vi "LogToStringControl.vi"(4 "Reduce By (0.2)":dbl=0.2, 5 "Clear":bool, 6 "Reduce Every (100)":i32=100, 7 "Enable":bool=TRUE, 8 "Time Stamp (T/F or Format)":variant=variant(bool FALSE), 9 "Prefix (\"\")":string, 10 "Log Text (\"\")":string, 11 "String Ref":refnum<vi>) -> (3 "String Ref out":refnum<vi>)   [LabVIEW 2021]
uses:
  <vilib>/regexp/Match Regular Expression.xnode
  <vilib>/Utility/Data Type/NI_Data Type.lvlib
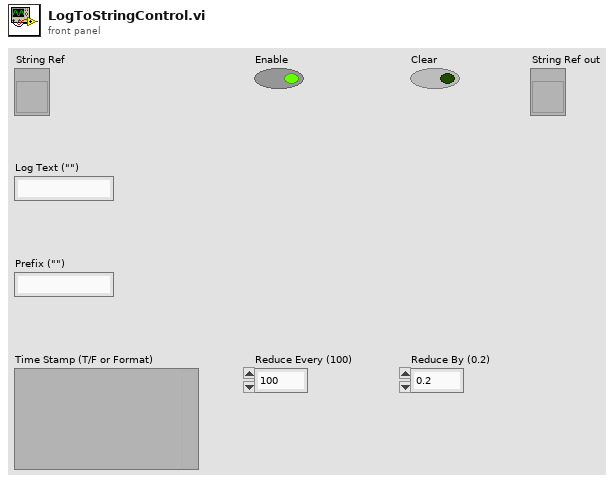
[diagram p1: front panel]
types:
  T1 = enum16{"Native", "Native Command Line", "UNIX", "Macintosh", "DOS"}
  T2 = typedef "NI_Data Type.lvlib/Data Type.ctl" = enum8{"Invalid Type", "Void", "I8", "I16", "I32", "I64", "U8", "U16", "U32", "U64", "Single Float", "Double Float", "Extended Float", "Single Complex", "Double Complex", "Extended Complex", "Enum U8", "Enum U16", "Enum U32", "Enum U64", "Single Float With Unit", "Double Float With Unit", "Extended Float With Unit", "Single Complex with Unit", "Double Complex with Unit", "Extended Complex with Unit", "Boolean", "String", "Path", "Picture", "Tag", "Array", "Cluster", "Variant", "LV Variant", "Waveform", "Timestamp", "Digital Waveform", "Digital Data", "ExpressData", "Refnum", "External Data", "VI", "Poly VI", "LabVIEW Class Instance", "Fixed Point", "Set Collection", "Map Collection"}
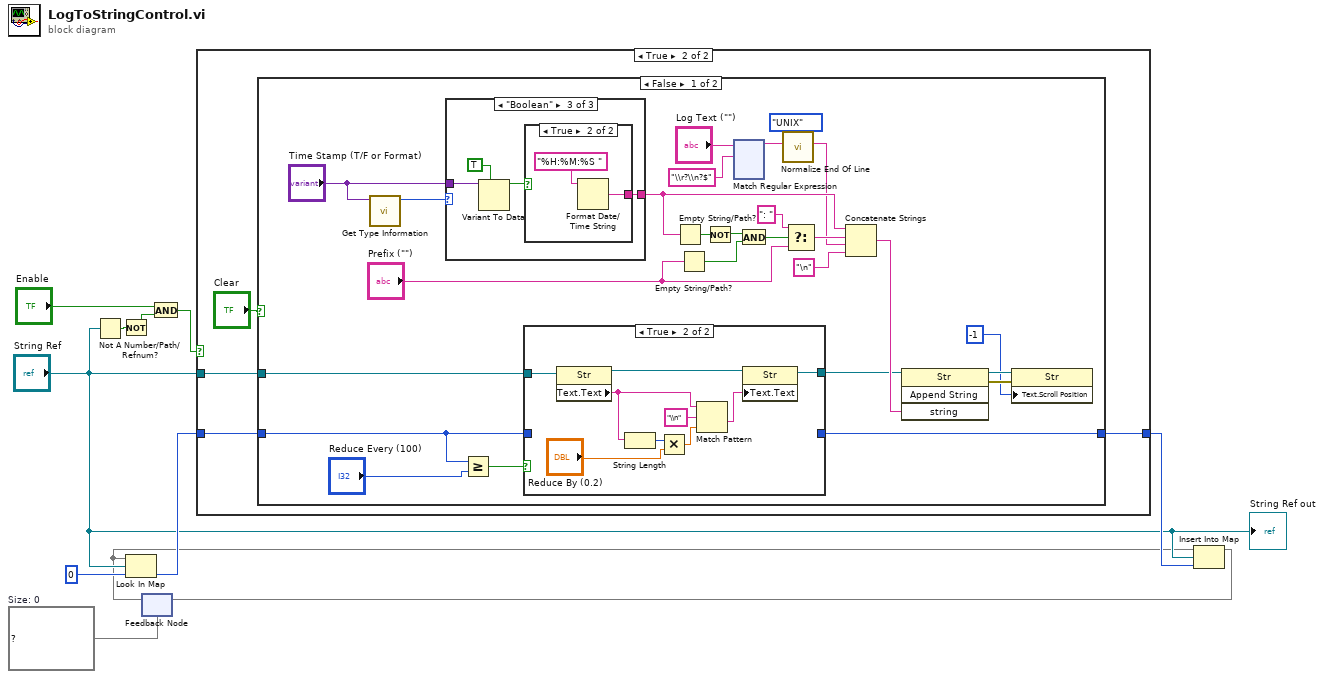
[diagram p0: block diagram]
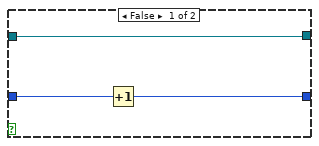
[diagram p3: hidden frame]
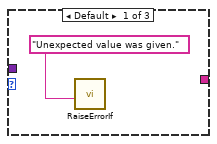
[diagram p4: hidden frame]
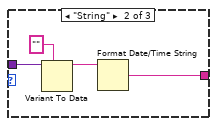
[diagram p5: hidden frame]
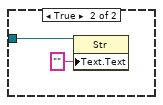
[diagram p7: hidden frame]
diagram:
  w7 = map{refnum<vi>, i32} {}  # Size: 0
  n1 = Not A Number/Path/Refnum?(number/path/refnum="String Ref") -> (NaN/Path/Refnum?=w10:bool)
  n2 = Not(x=w10) -> (.not. x?=w9:bool)
  n3 = feedback #1(w7) -> (w1:map{refnum<vi>, i32})
  n4 = Look In Map(map=w1, key="String Ref", default value=0) -> (value=w5:i32)  [unwired: 1 out]
  n5 = And(x="Enable", y=w9) -> (x .and. y?=w8:bool)
  n6 = case shown="True" w8 {
    tunnel: "String Ref" -> [_ w16]
    tunnel: w5 -> [w12 w15]
    tunnel: [w12 w14] -> w4
    frame False {
    }
    frame True {
      n7 = case shown="False" "Clear" {
        tunnel: w16 -> [w42 w184]
        tunnel: w15 -> [w26 _]
        tunnel: [w25 _] -> w14
        frame False {
          n8 = call <vilib>:"Get Type Information.vi"("variant"="Time Stamp (T/F or Format)") -> ("type"=w34:T2)  [unwired: 6 in, 4 out]
          n9 = case shown="\"Boolean\"" w34 {
            tunnel: "Time Stamp (T/F or Format)" -> [_ w175 w180]
            tunnel: [_ w173 w177] -> w40
            frame Default {
              n10 = call "RaiseErrorIf.vi"("error message"="Unexpected value was given.") -> ()  [unwired: 10 in, 1 out]
            }
            frame "String" {
              n11 = Variant To Data(type="" ("Log Text (\"\")"), Variant=w175) -> (data=w174:string)  [unwired: 1 in, 1 out]
              n12 = Format Date/Time String(time format string (%c)=w174) -> (date/time string=w173:string)  [unwired: 2 in]
            }
            frame "Boolean" {
              n13 = Variant To Data(type=TRUE, Variant=w180) -> (data=w178:bool)  [unwired: 1 in, 1 out]
              n14 = case shown="True" w178 {
                tunnel: [_ w181] -> w177
                frame False {
                }
                frame True {
                  n15 = Format Date/Time String(time format string (%c)="%H:%M:%S ") -> (date/time string=w181:string)  [unwired: 2 in]
                }
              }
            }
          }
          n16 = Greater Or Equal?(x=w26, y="Reduce Every (100)") -> (x >= y?=w32:bool)
          n17 = case shown="True" w32 {
            tunnel: w42 -> [w162 w171]
            tunnel: w26 -> [w161 _]
            tunnel: [w162 w163] -> w30
            tunnel: [w160 _] -> w25
            frame False {
              n18 = Increment(x=w161) -> (x+1=w160:i32)
            }
            frame True {
              n19 = property class="Str"(reference=w171) -> (reference out=w165:refnum<vi>, "Text.Text"=w166:string)  [unwired: 1 in, 1 out]
              n20 = String Length(string=w166) -> (length=w170:i32)
              n21 = Multiply(x=w170, y="Reduce By (0.2)") -> (x*y=w167:dbl)
              n22 = Match Pattern(string=w166, regular expression="\\n", offset (0)=w167) -> (after substring=w164:string)  [unwired: 3 out]
              n23 = property class="Str"(reference=w165, "Text.Text"=w164) -> (reference out=w163:refnum<vi>)  [unwired: 1 in, 1 out]
            }
          }
          n24 = Empty String/Path?(string/path=w40) -> (empty?=w35:bool)
          n25 = Empty String/Path?(string/path="Prefix (\"\")") -> (empty?=w39:bool)
          n26 = Not(x=w35) -> (.not. x?=w38:bool)
          n27 = xnode "Match Regular Expression"("input string"="Log Text (\"\")", "regular expression"="\\r?\\n?$") -> ("before match"=w18:string)  [unwired: 4 in, 4 out]
          n28 = And(x=w38, y=w39) -> (x .and. y?=w36:bool)
          n29 = call <vilib>:"Normalize End Of Line.vi"("end of line (Native)"=T1."UNIX", "string in"=w18) -> ("string out"=w22:string)  [unwired: 6 in]
          n30 = Select(t=": ", s=w36, f="Prefix (\"\")") -> (s? t:f=w41:string)
          n31 = Concatenate Strings(w40, w41, w22, "\n" ("string")) -> (w31:string)
          n32 = invoke class="Str" method="Append String"(reference=w30, "string"=w31) -> (reference out=w29:refnum<vi>, error out=w28:errorcluster)  [unwired: 2 in, 2 out]
          n33 = property class="Str"(reference=w29, error in=w28, "Text.Scroll Position"=-1) -> ()  [unwired: 2 out]
        }
        frame True {
          n34 = property class="Str"(reference=w184, "Text.Text"="") -> ()  [unwired: 1 in, 2 out]
        }
      }
    }
  }
  n35 = Insert Into Map(map in=w1, key="String Ref", value=w4) -> (map out=w2:map{refnum<vi>, i32})  [unwired: 2 out]
  n36 = feedback-in #1(w2) -> ()
  "String Ref out" <- "String Ref"
